vi "Scope AWG Loopback.vi"() -> ()   [LabVIEW 2023]
uses:
  <instrlib>/niFgen/niFgen.llb/niFgen Output Mode.ctl
  <instrlib>/niScope/Controls/niScope trigger source digital.ctl
  <instrlib>/niScope/Controls/niScope trigger slope.ctl
  <instrlib>/niScope/Controls/niScope vertical coupling.ctl
  <instrlib>/niFgen/niFgen.llb/niFgen_ctl Exported Signal Desination Values (ComboBox).ctl
  <instrlib>/niFgen/niFgen.llb/niFgen_ctl Exported Signal Name Values (Ring).ctl
  <instrlib>/niFgen/niFgen.llb/niFgen_ctl Exported Signal Identifiers (Ring).ctl
  <instrlib>/niScope/Configure/Trigger/niScope Configure Trigger Digital.vi
  <instrlib>/niScope/Measurements/niScope Multi Fetch Array Measurement Cluster.vi
  <instrlib>/niFgen/niFgen.llb/niFgen Write Waveform.vi
panel:
  in  "Stimulus":enum32{"Custom Sin like", "Control"}(tab)
  in  "Sequence":T1(array[cluster])=[{"Waveform Name"=0, "# Loops"=1, "Marker"=-1}, {"Waveform Name"=1, "# Loops"=1, "Marker"=-1}, {"Waveform Name"=2, "# Loops"=3, "Marker"=-1}, {"Waveform Name"=3, "# Loops"=1, "Marker"=-1}] {"Waveform Name" items=["0: Big Ramp", "1: Small Sine", "2: Half Sized Square", "3: DC 0V"]}
  in  "Waveform Array":T2(array[cluster])=[{"Name"="Big Ramp", "Waveform"={"Waveform Type"=5, "Amplitude"=1.0, "# of points"=256}}, {"Name"="Small Sine", "Waveform"={"Waveform Type"=0, "Amplitude"=0.5, "# of points"=256}}, {"Name"="Half Sized Square", "Waveform"={"Waveform Type"=3, "Amplitude"=0.5, "# of points"=256}}, {"Name"="DC 0V", "Waveform"={"Waveform Type"=7, "Amplitude"=0.0, "# of points"=256}}] caption="Waveform Information Array" {"Waveform"."Amplitude" min=0.0 max=1.0 format="%.2f"; "Waveform"."Waveform Type" items=["Sine", "Cosine", "Triangle", "Square", "Sawtooth", "Increasing Ramp", "Decreasing Ramp", "DC Value"]}
  in  "reference position":dbl=50.0 format="%#_13g"
  out "Waveform Target":dbl[][](graph)
  out "error out":errorcluster
  in  "Scope record length":i32=1000 caption="min record length"
  in  "Scope sample rate":dbl=20000000.0 caption="min sample rate" format="%^.2e"
  in  "Scope channels":string="1"
  in  "AWG Name":refnum<k15>="AWG_5433_C02_S04"
  in  "Scope name":refnum<k15>="Scope_5152_C02_S05"
  out "Waveform Graph":T3(graph)
  in  "Stop":bool
  in  "AWG Channels":string="0"
  in  "DC Offset":dbl format="%.4f"
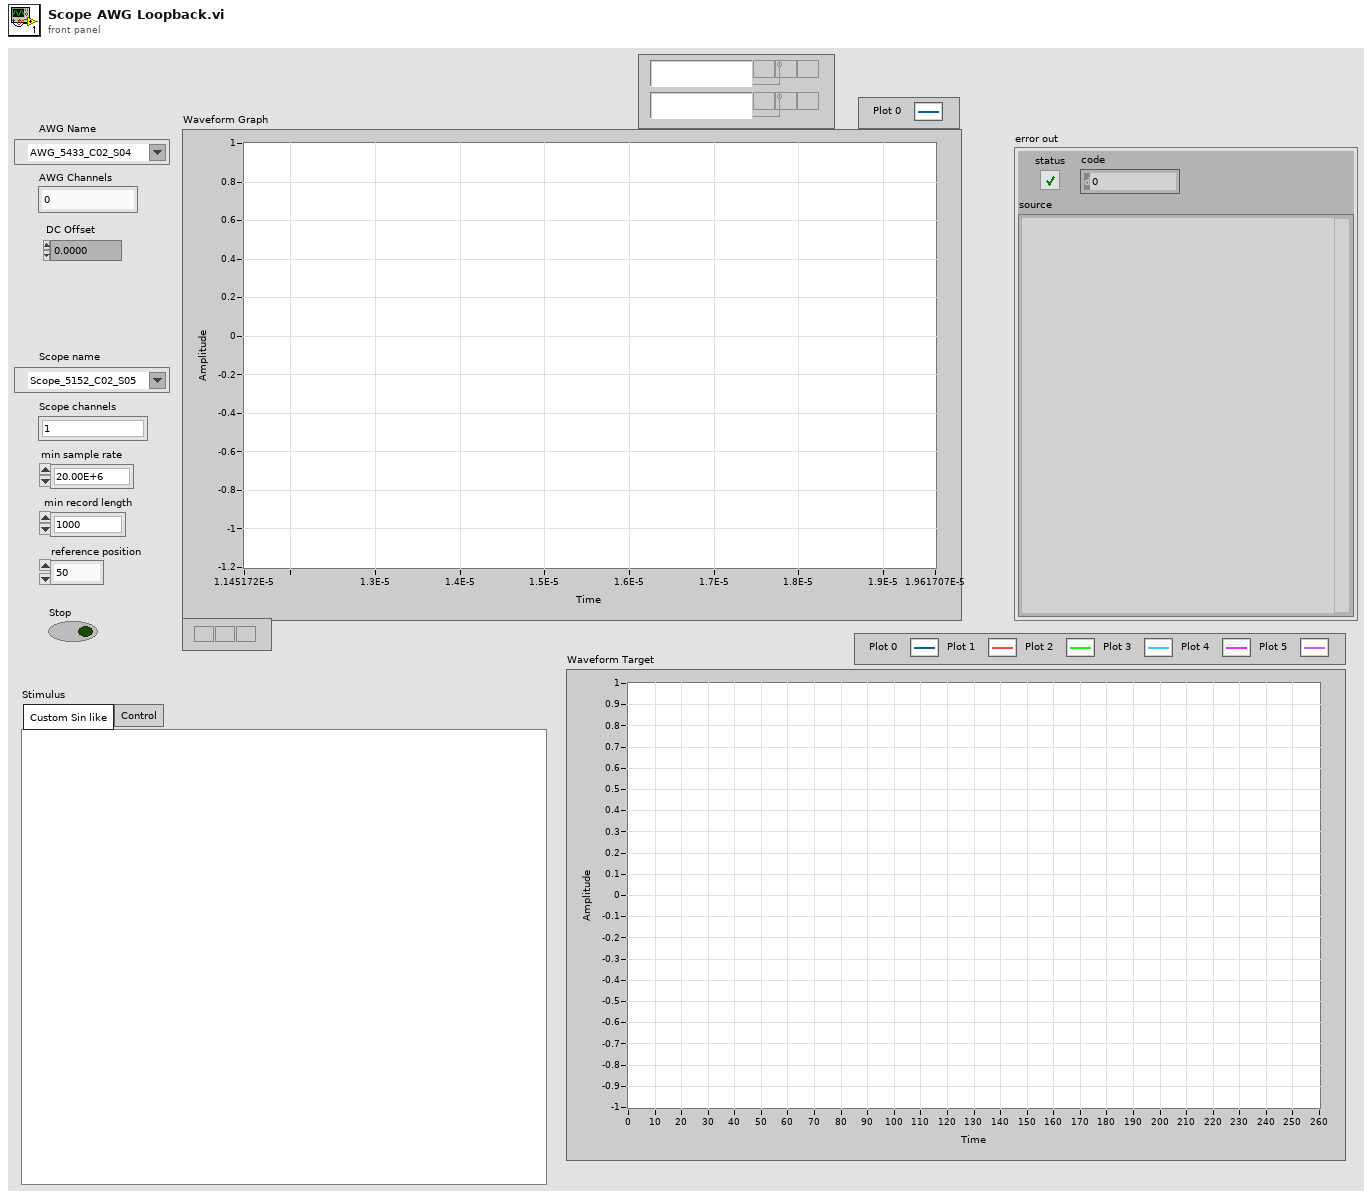
[diagram p1: front panel]
types:
  T1 = cluster{"Waveform Name":u16, "# Loops":i32, "Marker":i32}[]
  T2 = cluster{"Name":string, "Waveform":cluster{"Waveform Type":u16, "Amplitude":dbl, "# of points":u32}}[]
  T3 = cluster{"relativeInitialX":dbl, "xIncrement":dbl, "measWfm":dbl[]}[]
  T4 = typedef "niFgen_ctl Exported Signal Identifiers (Ring).ctl" = string
  T5 = typedef "niFgen_ctl Exported Signal Name Values (Ring).ctl" = u16
  T6 = typedef "niFgen_ctl Exported Signal Desination Values (ComboBox).ctl" = string
  T7 = typedef "niScope vertical coupling.ctl" = i32
  T8 = typedef "niScope trigger slope.ctl" = i32
  T9 = typedef "niScope trigger source digital.ctl" = string
  T10 = typedef "niFgen Output Mode.ctl" = u32
  T11 = cluster{"Waveform Type":u16, "Amplitude":dbl, "# of points":u32}
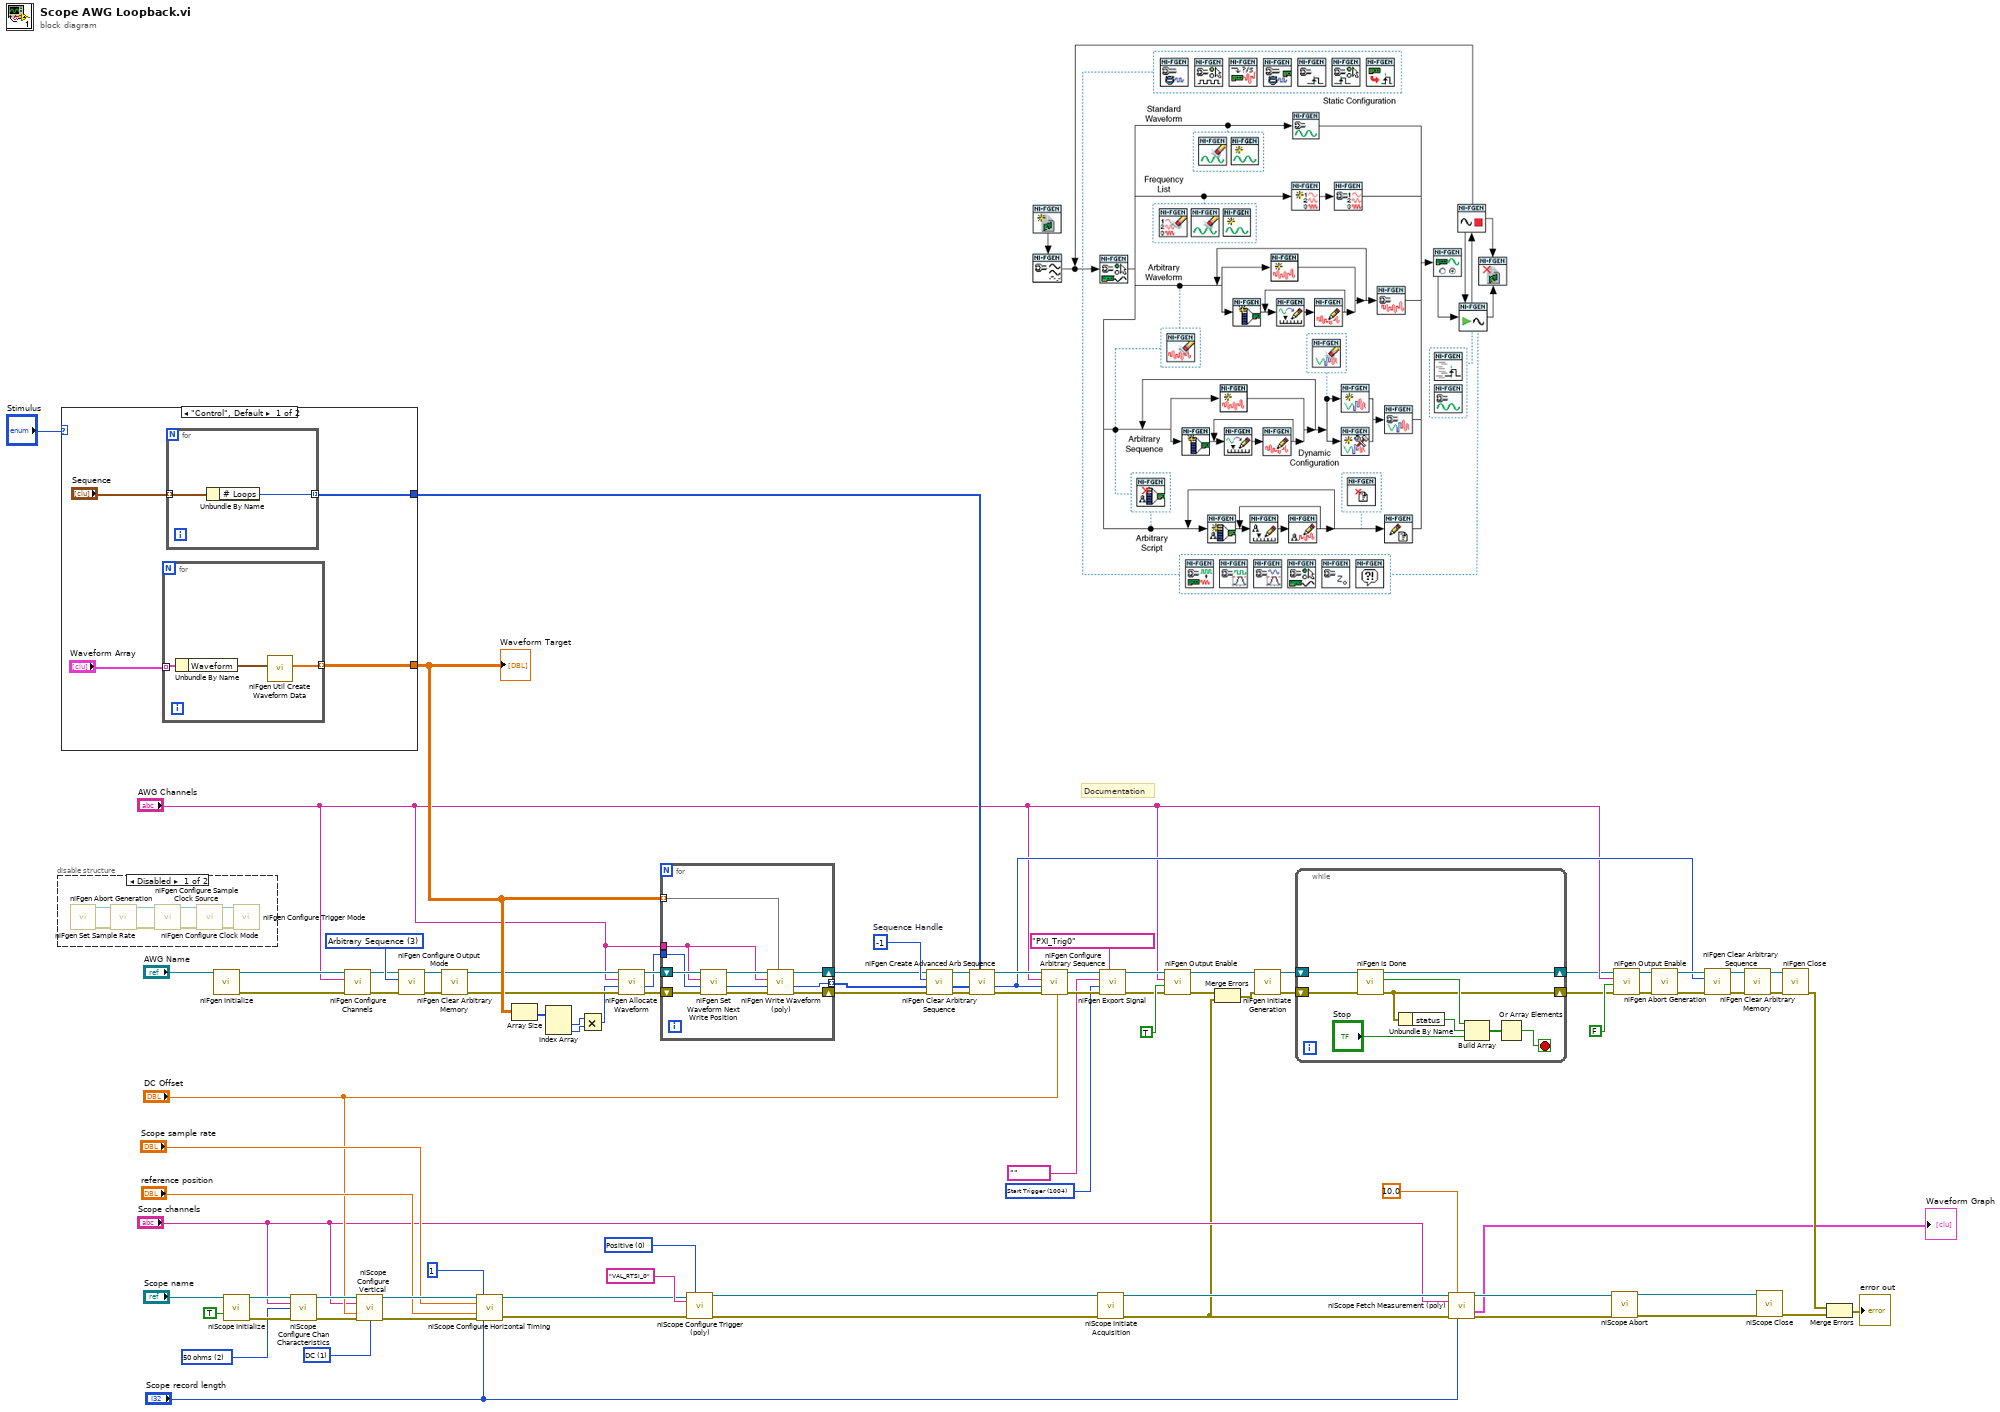
[diagram p0: block diagram]
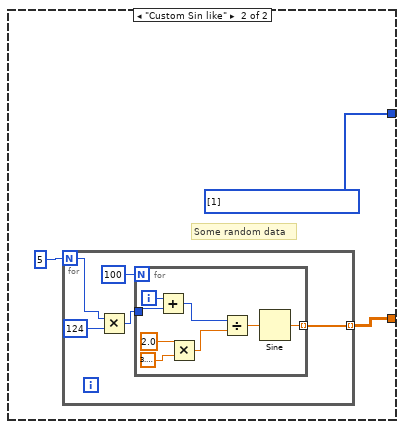
[diagram p2: hidden frame]
diagram:
  w22 = -1  # Sequence Handle
  w43 = T5 1004 items=["Sample Clock"=101, "Sample Clock Timebase"=1006, "Reference Clock"=102, "Onboard Reference Clock"=1019, "Start Trigger"=1004, "Script Trigger"=103, "Marker Event"=1001, "Data Marker Event"=108, "Ready For Start Event"=105, "Started Event"=106, "Done Event"=107, "Synchronization Pulse"=1007, "Sync Out"=1002] ("Signal")
  w56 = T7 1 items=["AC", "DC", "Ground"] ("vertical coupling")
  w63 = T8 0 items=["Positive", "Negative"] ("trigger slope")
  w66 = u32 2 items=["1 mega ohm"=0, "50 ohms"=2] ("input impedance")
  w85 = T10 3 items=["Standard Function", "Frequency List", "Arbitrary Waveform", "Arbitrary Sequence", "Script"] ("Output Mode (default: 0=Standard Function)")
  # "Documentation"
  n1 = disable-structure shown="Disabled" {
    frame Disabled {
      n2 = call <instrlib>:"niFgen Abort Generation.vi"() -> ("error out"=w92:errorcluster, "Instrument Handle Out"=w93:refnum<k15>)  [unwired: 10 in]
      n3 = call <instrlib>:"niFgen Set Sample Rate.vi"("error in (no error)"=w92, "Instrument Handle"=w93) -> ("error out"=w91:errorcluster, "Instrument Handle Out"=w88:refnum<k15>)  [unwired: 8 in]
      n4 = call <instrlib>:"niFgen Configure Sample Clock Source.vi"("error in (no error)"=w91, "Instrument Handle"=w88) -> ("error out"=w90:errorcluster, "Instrument Handle Out"=w89:refnum<k15>)  [unwired: 8 in]
      n5 = call <instrlib>:"niFgen Configure Clock Mode.vi"("error in (no error)"=w90, "Instrument Handle"=w89) -> ("error out"=w94:errorcluster, "Instrument Handle Out"=w95:refnum<k15>)  [unwired: 8 in]
      n6 = call <instrlib>:"niFgen Configure Trigger Mode.vi"("error in (no error)"=w94, "Instrument Handle"=w95) -> ()  [unwired: 8 in, 2 out]
    }
    frame Enabled {
    }
  }
  n7 = case shown="\"Control\", Default" "Stimulus" {
    tunnel: [w98 w107] -> w48
    tunnel: [w96 i32[] [1] ("Loop Counts Array")] -> w16
    frame "Control", Default {
      n8 = for {
        tunnel: "Waveform Array" -> [w104] mode=indexing
        tunnel: [w102] -> w98 mode=indexing
        n9 = Unbundle By Name(w104) -> ("Waveform"=w103:T11)
        n10 = call <instrlib>:"niFgen Util Create Waveform Data.vi"("Waveform"=w103) -> ("Waveform Data"=w102:dbl[])  [unwired: 10 in]
      }
      n11 = for {
        tunnel: "Sequence" -> [w101] mode=indexing
        tunnel: [w100] -> w96 mode=indexing
        n12 = Unbundle By Name(w101) -> ("# Loops"=w100:i32)
      }
    }
    frame "Custom Sin like" {
      # "Some random data"
      n13 = for {
        N: 5 -> [w110]
        tunnel: [w111] -> w107 mode=indexing
        n14 = Multiply(x=w110, y=124) -> (x*y=w108:i32)
        n15 = for {
          N: 100 -> [_]
          tunnel: [w120] -> w111 mode=indexing
          tunnel: w108 -> [w115]
          i -> [w116]
          n16 = Add(x=w116, y=w115) -> (x+y=w114:i32)
          n17 = Multiply(x=2.0, y=3.141592653589793) -> (x*y=w119:dbl)
          n18 = Divide(x=w114, y=w119) -> (x/y=w113:dbl)
          n19 = Sine(x=w113) -> (sin(x)=w120:dbl)
        }
      }
    }
  }
  "Waveform Target" <- w48
  n20 = call <instrlib>:"niFgen Initialize.vi"("Resource Name"="AWG Name") -> ("error out"=w28:errorcluster, "Instrument Handle Out"=w29:refnum<k15>)  [unwired: 9 in]
  n21 = call <instrlib>:"niScope Initialize.vi"("resource name"="Scope name", "reset device"=TRUE) -> ("instrument handle"=w68:refnum<k15>, "error out"=w69:errorcluster)  [unwired: 12 in]
  n22 = call <instrlib>:"niScope Configure Chan Characteristics.vi"("instrument handle"=w68, "channels"="Scope channels", "input impedance"=w66, "error in"=w69) -> ("instrument handle out"=w67:refnum<k15>, "error out"=w55:errorcluster)  [unwired: 10 in]
  n23 = call <instrlib>:"niFgen Configure Channels.vi"("error in (no error)"=w28, "Channels"="AWG Channels", "Instrument Handle"=w29) -> ("error out"=w84:errorcluster, "Instrument Handle Out"=w83:refnum<k15>)  [unwired: 7 in]
  n24 = call <instrlib>:"niScope Configure Vertical.vi"("instrument handle"=w67, "vertical coupling"=w56, "channels"="Scope channels", "vertical offset"="DC Offset", "error in"=w55) -> ("instrument handle out"=w73:refnum<k15>, "error out"=w75:errorcluster)  [unwired: 9 in]
  n25 = call <instrlib>:"niFgen Configure Output Mode.vi"("error in (no error)"=w84, "Output Mode (default: 0=Standard Function)"=w85, "Instrument Handle"=w83) -> ("error out"=w32:errorcluster, "Instrument Handle Out"=w31:refnum<k15>)  [unwired: 6 in]
  n26 = call <instrlib>:"niFgen Clear Arbitrary Memory.vi"("error in (no error)"=w32, "Instrument Handle"=w31) -> ("error out"=w33:errorcluster, "Instrument Handle Out"=w30:refnum<k15>)  [unwired: 8 in]
  n27 = call <instrlib>:"niScope Configure Horizontal Timing.vi"("instrument handle"=w73, "number of records"=1, "min sample rate"="Scope sample rate", "reference position"="reference position", "error in"=w75, "min record length"="Scope record length") -> ("instrument handle out"=w72:refnum<k15>, "error out"=w74:errorcluster)  [unwired: 8 in]
  n28 = Array Size(array=w48) -> (size(s)=w4:i32[])
  n29 = Index Array(array=w4) -> (element #1=w3:i32, element #2=w2:i32)  [unwired: 2 in]
  n30 = Multiply(x=w3, y=w2) -> (x*y=w1:i32)
  n31 = call <instrlib>:"niFgen Allocate Waveform.vi"("error in (no error)"=w33, "Waveform Size"=w1, "Channel Name"="AWG Channels", "Instrument Handle"=w30) -> ("error out"=w7:errorcluster, "Waveform Handle Out"=w5:i32, "Instrument Handle Out"=w6:refnum<k15>)  [unwired: 5 in]
  n32 = for {
    shift-right: [w129] -> w21
    shift-left: w7 -> [w131]
    shift-right: [w126] -> w20
    shift-left: w6 -> [w128]
    tunnel: "AWG Channels" -> [w125]
    tunnel: w5 -> [w124]
    tunnel: [w123] -> w52 mode=indexing
    tunnel: w48 -> [w121] mode=indexing
    n33 = call <instrlib>:"niFgen Set Waveform Next Write Position.vi"("error in (no error)"=w131, "Waveform Handle"=w124, "Channel Name"=w125, "Instrument Handle"=w128) -> ("error out"=w130:errorcluster, "Waveform Handle Out"=w122:i32, "Instrument Handle Out"=w127:refnum<k15>)  [unwired: 5 in]
    n34 = call-poly <instrlib>:"niFgen Write Waveform (poly).vi"("Waveform Data"=w121, "error in (no error)"=w130, "Waveform Handle"=w122, "Channel Name"=w125, "Instrument Handle"=w127) -> ("error out"=w129:errorcluster, "Waveform Handle Out"=w123:i32, "Instrument Handle Out"=w126:refnum<k15>)  [unwired: 4 in]
  }
  n35 = call-poly <instrlib>:"niScope Configure Trigger (poly).vi"("instrument handle"=w72, "trigger slope"=w63, "trigger source"=T9 "VAL_RTSI_0", "error in"=w74) -> ("instrument handle out"=w80:refnum<k15>, "error out"=w79:errorcluster)  [unwired: 10 in]
  n36 = call <instrlib>:"niFgen Clear Arbitrary Sequence.vi"("error in (no error)"=w21, "Sequence Handle"=w22, "Instrument Handle"=w20) -> ("error out"=w19:errorcluster, "Instrument Handle Out"=w18:refnum<k15>)  [unwired: 7 in]
  n37 = call <instrlib>:"niFgen Create Advanced Arb Sequence.vi"("Loop Counts Array"=w16, "error in (no error)"=w19, "Waveform Handles Array"=w52, "Instrument Handle"=w18) -> ("error out"=w54:errorcluster, "Sequence Handle"=w51:i32, "Instrument Handle Out"=w53:refnum<k15>)  [unwired: 4 in, 1 out]
  n38 = call <instrlib>:"niFgen Configure Arbitrary Sequence.vi"("Offset"="DC Offset", "error in (no error)"=w54, "Sequence Handle"=w51, "Channel Name"="AWG Channels", "Instrument Handle"=w53) -> ("error out"=w45:errorcluster, "Instrument Handle Out"=w46:refnum<k15>)  [unwired: 5 in]
  n39 = call <instrlib>:"niScope Initiate Acquisition.vi"("instrument handle"=w80, "error in"=w79) -> ("instrument handle out"=w41:refnum<k15>, "error out"=w39:errorcluster)  [unwired: 12 in]
  n40 = call <instrlib>:"niFgen Export Signal.vi"("Output Terminal (do not export)"=T6 "PXI_Trig0", "error in (no error)"=w45, "Signal"=w43, "Signal Identifier (None)"=T4 "", "Instrument Handle"=w46) -> ("error out"=w25:errorcluster, "Instrument Handle Out"=w26:refnum<k15>)  [unwired: 5 in]
  n41 = call <instrlib>:"niFgen Output Enable.vi"("error in (no error)"=w25, "Output Enable (default: True)"=TRUE ("output enable"), "Channel Name"="AWG Channels", "Instrument Handle"=w26) -> ("error out"=w23:errorcluster, "Instrument Handle Out"=w24:refnum<k15>)  [unwired: 6 in]
  n42 = Merge Errors(w23, w39) -> (w61:errorcluster)
  n43 = call <instrlib>:"niFgen Initiate Generation.vi"("error in (no error)"=w61, "Instrument Handle"=w24) -> ("error out"=w82:errorcluster, "Instrument Handle Out"=w81:refnum<k15>)  [unwired: 8 in]
  n44 = while {
    shift-right: [w134] -> w13
    shift-left: w82 -> [w133]
    shift-right: [w135] -> w12
    shift-left: w81 -> [w132]
    stop <- w140 stop-if-true
    n45 = call <instrlib>:"niFgen Is Done.vi"("error in (no error)"=w133, "Instrument Handle"=w132) -> ("error out"=w134:errorcluster, "Done"=w136:bool, "Instrument Handle Out"=w135:refnum<k15>)  [unwired: 7 in]
    n46 = Unbundle By Name(w134) -> ("status"=w137:bool)
    n47 = Build Array(w136, w137, "Stop") -> (w138:bool[])
    n48 = Or Array Elements(Boolean array=w138) -> (logical OR=w140:bool)
  }
  n49 = call-poly <instrlib>:"niScope Fetch Measurement (poly).vi"("instrument handle"=w41, "timeout"=10.0, "channels"="Scope channels", "error in"=w39, "meas waveform size"="Scope record length") -> ("instrument handle out"=w38:refnum<k15>, "meas waveform"=→"Waveform Graph":T3, "error out"=w36:errorcluster)  [unwired: 7 in, 1 out]
  n50 = call <instrlib>:"niScope Abort.vi"("instrument handle"=w38, "error in"=w36) -> ("instrument handle out"=w78:refnum<k15>, "error out"=w77:errorcluster)  [unwired: 12 in]
  n51 = call <instrlib>:"niFgen Output Enable.vi"("error in (no error)"=w13, "Output Enable (default: True)"=FALSE ("output enable"), "Channel Name"="AWG Channels", "Instrument Handle"=w12) -> ("error out"=w10:errorcluster, "Instrument Handle Out"=w11:refnum<k15>)  [unwired: 6 in]
  n52 = call <instrlib>:"niFgen Abort Generation.vi"("error in (no error)"=w10, "Instrument Handle"=w11) -> ("error out"=w87:errorcluster, "Instrument Handle Out"=w86:refnum<k15>)  [unwired: 8 in]
  n53 = call <instrlib>:"niFgen Clear Arbitrary Sequence.vi"("error in (no error)"=w87, "Sequence Handle"=w51, "Instrument Handle"=w86) -> ("error out"=w8:errorcluster, "Instrument Handle Out"=w9:refnum<k15>)  [unwired: 7 in]
  n54 = call <instrlib>:"niFgen Clear Arbitrary Memory.vi"("error in (no error)"=w8, "Instrument Handle"=w9) -> ("error out"=w50:errorcluster, "Instrument Handle Out"=w49:refnum<k15>)  [unwired: 8 in]
  n55 = call <instrlib>:"niScope Close.vi"("instrument handle"=w78, "error in"=w77) -> ("error out"=w60:errorcluster)  [unwired: 13 in]
  n56 = call <instrlib>:"niFgen Close.vi"("error in (no error)"=w50, "Instrument Handle"=w49) -> ("error out"=w59:errorcluster)  [unwired: 9 in]
  n57 = Merge Errors(w59, w60) -> (→"error out":errorcluster)
